vi "Blank HMI Template.vi"() -> ()   [LabVIEW 2018]
uses:
  <vilib>/NI/STM/TCP/Read Meta Data (TCP Ref).vi
  <vilib>/NI/STM/TCP/Get Connection Reference (TCP).vi
  <vilib>/NI/AMC/Read Termination Message.vi
  <vilib>/NI/AMC/Create Single Message.vi
  <vilib>/NI/AMC/Update Message Routing Info.vi
  <vilib>/NI/STM/TCP/Read Meta Data (TCP Clst).vi
  <vilib>/NI/AMC/Globals.vi
  <vilib>/NI/AMC/Send Message.vi
  <vilib>/NI/AMC/AMC.lvlib
  <vilib>/NI/STM/NI STM.lvlib
panel:
  in  "Machine":bool
  in  "Basement 4":bool
  in  "Dryer":bool
  in  "Rinse 4":bool
  in  "Rinse 3":bool
  in  "Rinse 2":bool
  in  "Basement 3":bool
  in  "Basement 2":bool
  in  "Basement 1":bool
  in  "Plater 6":bool
  in  "Plater 5":bool
  in  "Plater 4":bool
  in  "Plater 3":bool
  in  "Plater 2":bool
  in  "Plater 1":bool
  in  "Predip":bool
  in  "Rinse 1":bool
  in  "Cleaner":bool
  in  "Loader":bool
  out "status":string
  # "Module Selection"
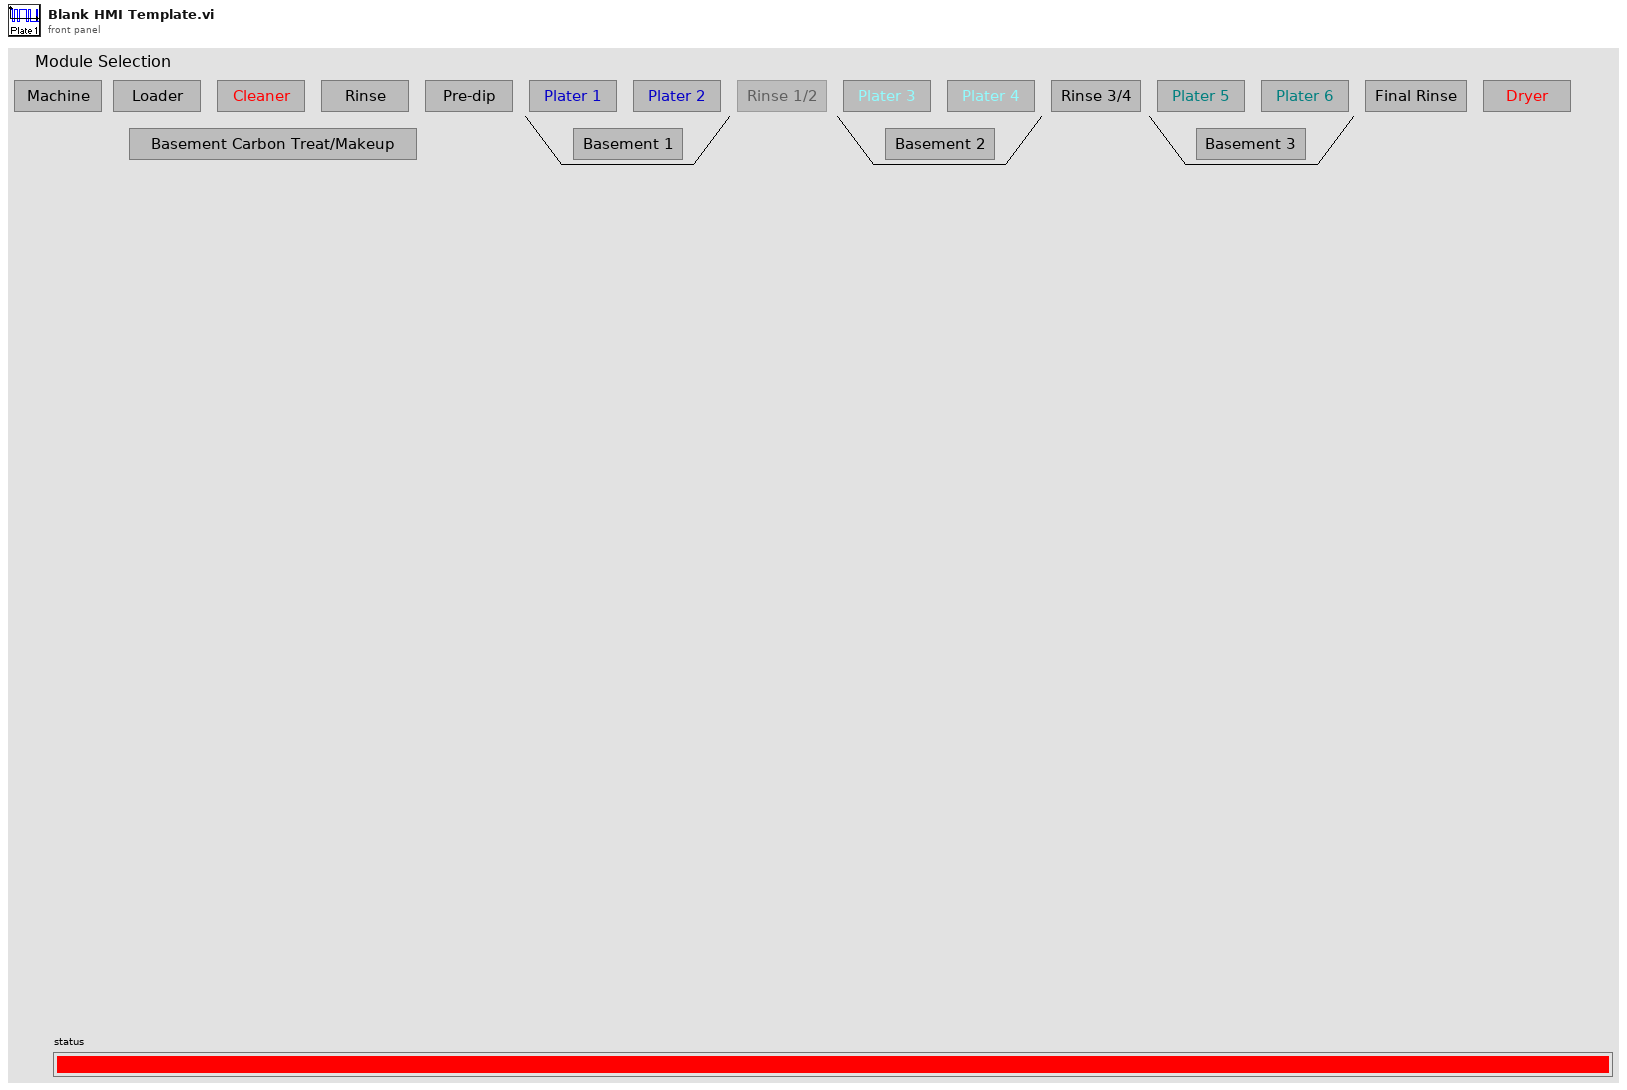
[diagram p1: front panel]
types:
  T1 = typedef "NI STM.lvlib/TCP Connection Info.ctl" = cluster{"connection ID":refnum<k5>, "meta data":T2[]}
  T2 = typedef "NI STM.lvlib/MetaDataElement.ctl" = string
  T3 = typedef "AMC.lvlib/Message Queue.ctl" = refnum<queue>
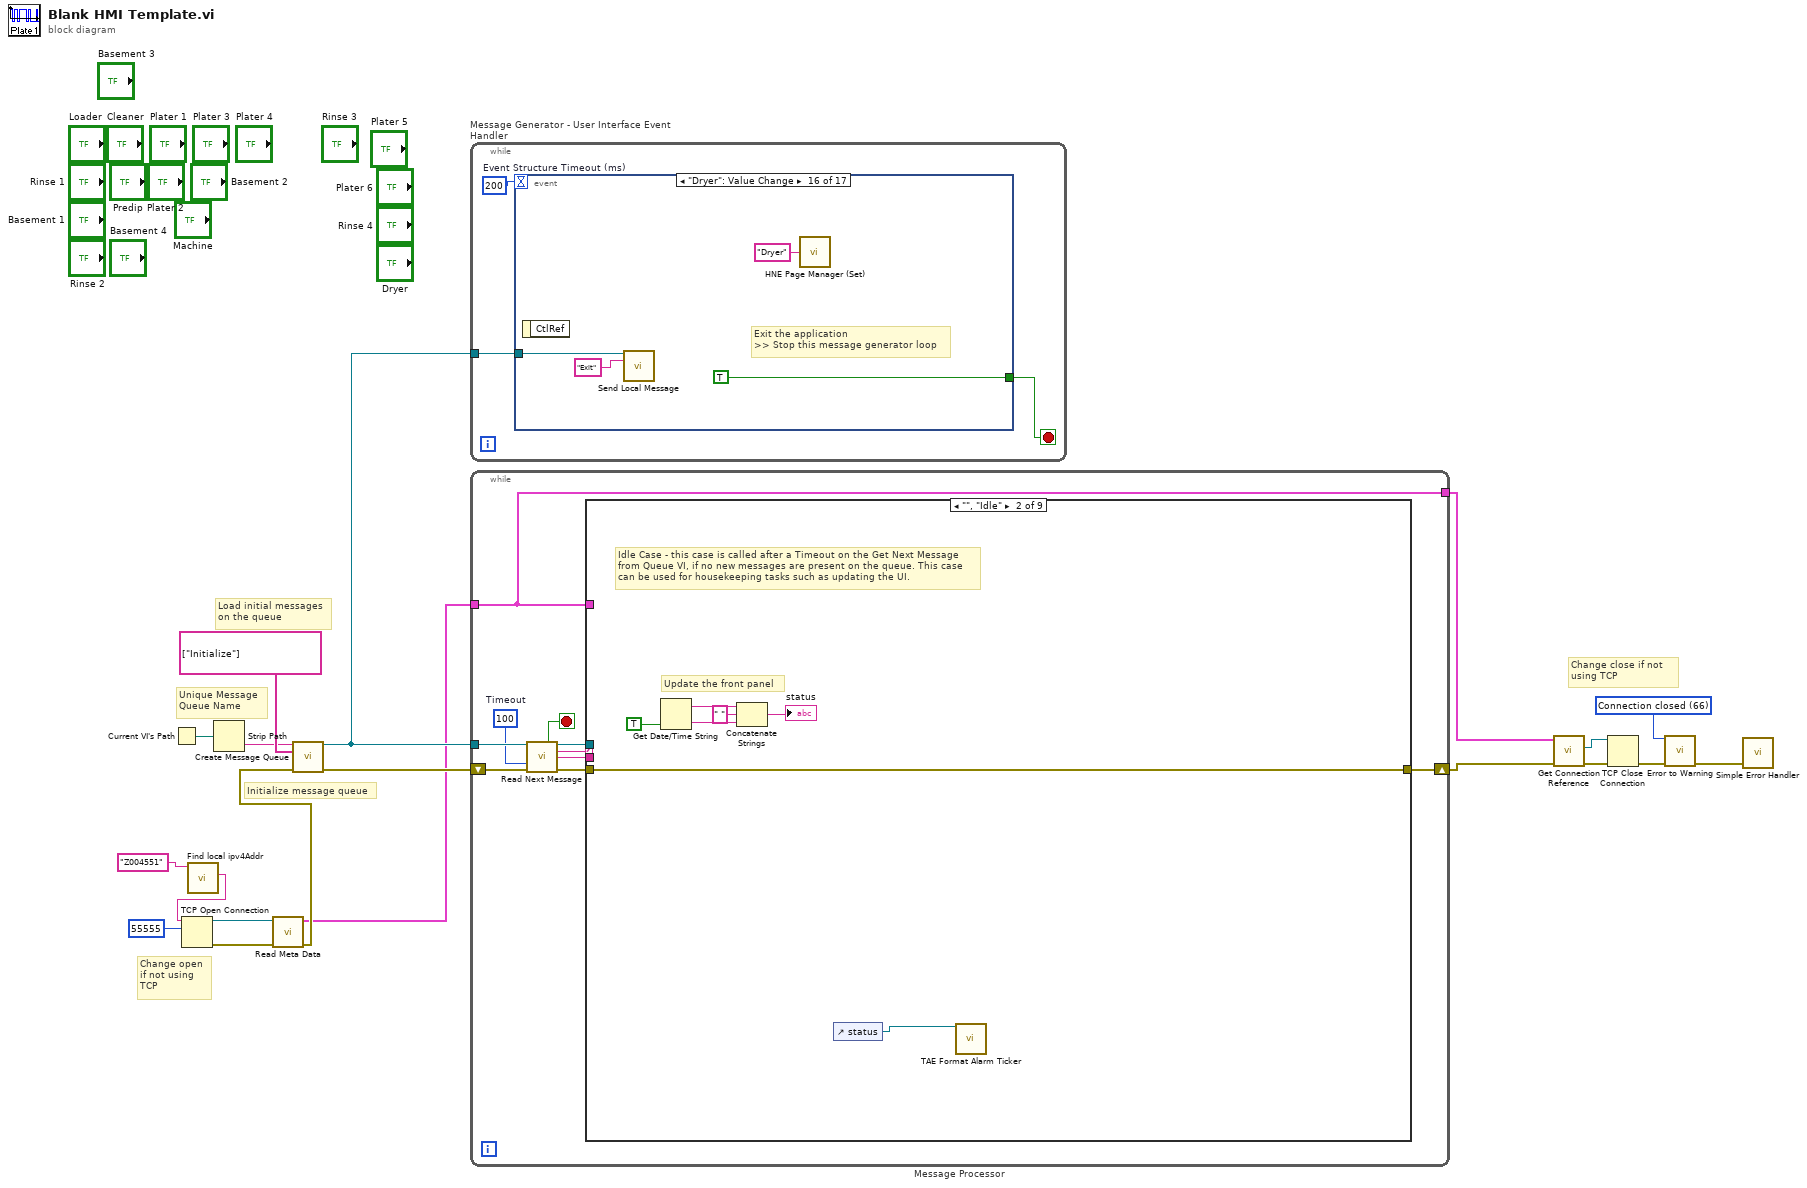
[diagram p0: block diagram]
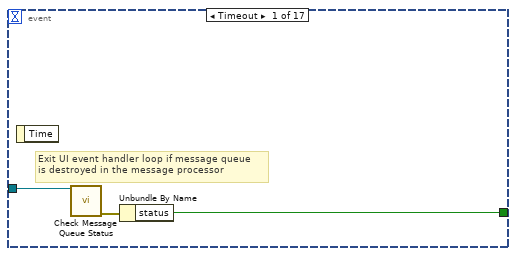
[diagram p2: hidden frame]
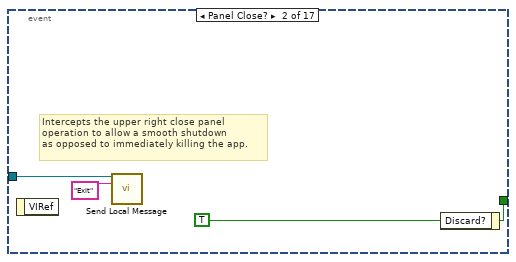
[diagram p3: hidden frame]
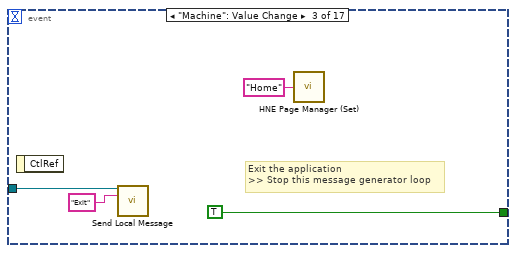
[diagram p4: hidden frame]
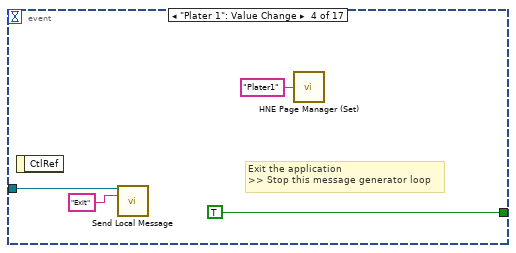
[diagram p5: hidden frame]
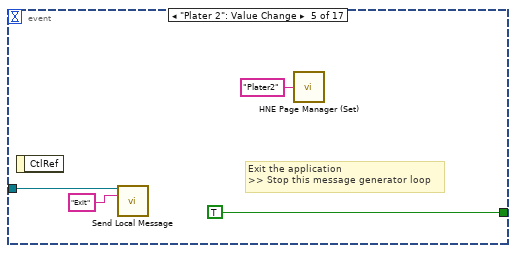
[diagram p6: hidden frame]
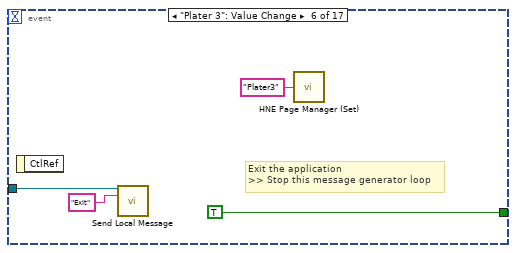
[diagram p7: hidden frame]
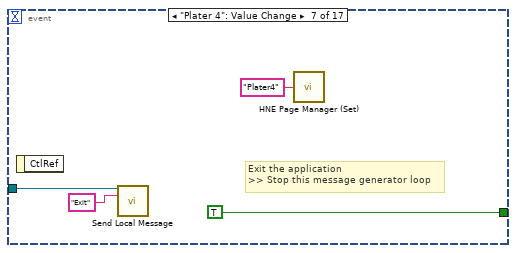
[diagram p8: hidden frame]
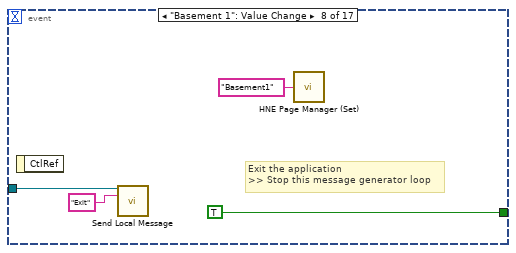
[diagram p9: hidden frame]
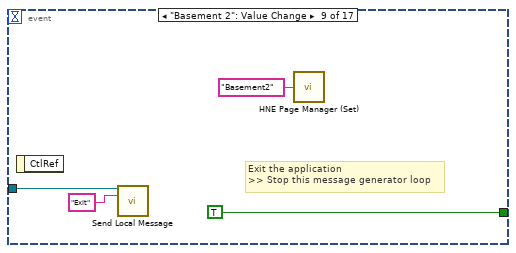
[diagram p10: hidden frame]
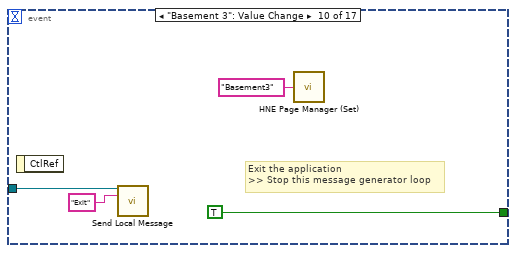
[diagram p11: hidden frame]
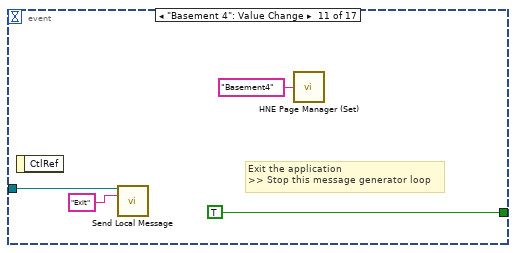
[diagram p12: hidden frame]
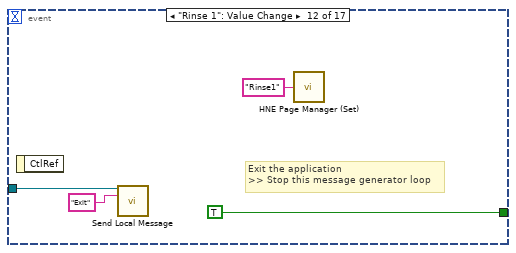
[diagram p13: hidden frame]
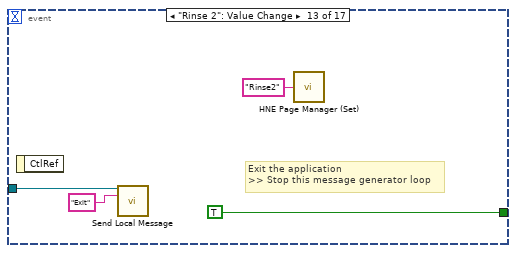
[diagram p14: hidden frame]
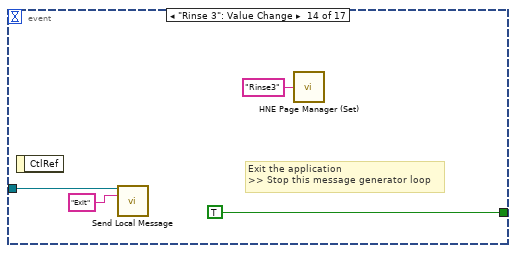
[diagram p15: hidden frame]
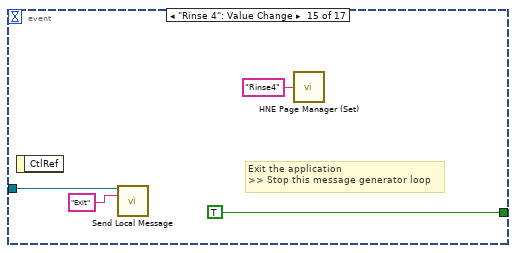
[diagram p16: hidden frame]
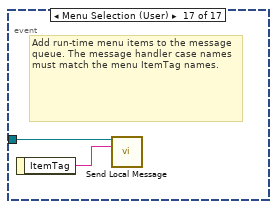
[diagram p17: hidden frame]
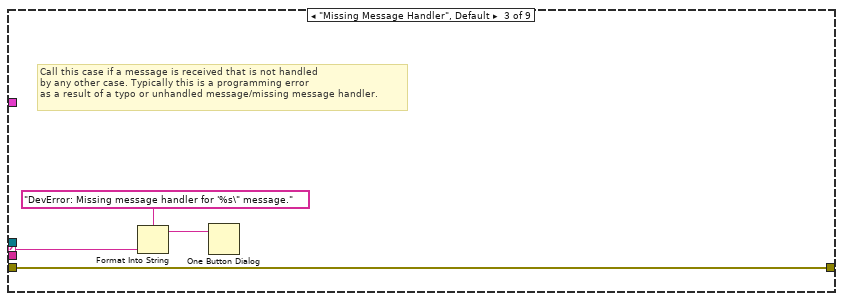
[diagram p19: hidden frame]
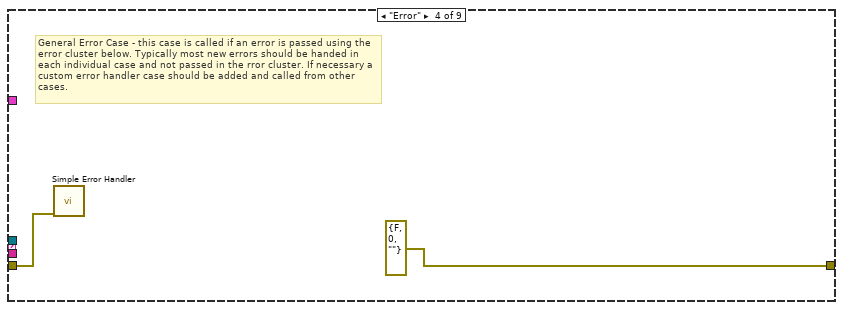
[diagram p20: hidden frame]
diagram:
  w8 = 66 items=["No Error", "Argument Error", "Memory Full", "Out of Zone", "End of File", "File Already Open", "Generic File IO Error", "File Not Found", "File Permission Error", "Disk Full", "Duplicate Path", "Too Many Files Open", "Not Enabled", "Resource File Not Found", "Cannot Add Resource", "Resource Not Found", "Image Not Found", "Image Memory Error", "Pen Does Not Exist", "Config Bad Type", "Config Token Not Found", "Config Parse Error", "Config Memory Error", "Bad External Code Format", "Bad External Code Offset", "External Code Not Present", "Null Window", "Destroy Window Mixup", "Null Menu", "Print Aborted", "Bad Print Record", "Print Driver Error", "Windows Error During Print", "Memory Error During Print", "Print Dialog Error", "Generic Print Error", "Invalid Device Refnum", "Device Not Found", "Device Parameter Error", "Device Unit Error", "Can't Open Device", "Device Call Aborted", "Generic Error", "Cancelled By User", "Object ID Too Low", "Object ID Too High", "Object Not In Heap", "Unknown Heap", "Bad DefProc ID", "DefProc Not In Table", "Message Out Of Range", "Null Method", "Unknown Message", "Manager Call Not Supported", "Bad address", "Connection In progress", "Connection timed out", "Connection is already in progress", "Network attribute not supported", "Network error", "Address in use", "System out of memory", "Connection aborted", "Connection refused", "Connection is not connected", "Connection is already connected", "Connection closed", "Initialize error (interapplication manager)", "Bad occurrence", "Wait on unbound occurrence handler", "Occurrence queue overflow", "Bad path", "Semaphore not signaled", "Unrecognized type (interapplication manager)"] ("1st Error to Convert")
  # "Change close if not using TCP"
  # "Change open if not using TCP"
  # "Initialize message queue"
  # "Unique Message\nQueue Name"
  # "Load initial messages\non the queue"
  n1 = Current VI's Path() -> (path=w15:path)
  n2 = call "Find local ipv4Addr.vi"("MachineToFind"="Z004551" ("Target IP Address")) -> ("name"=w1:string)  [unwired: 9 in, 1 out]
  n3 = TCP Open Connection(address=w1, remote port or service name=u16 55555 ("remote port")) -> (connection ID=w13:refnum<k5>, error out=w12:errorcluster)  [unwired: 1 in, 2 out]
  n4 = Strip Path(path=w15) -> (name=w18:string)  [unwired: 1 out]
  n5 = call-poly <vilib>:"Read Meta Data.vi"("error in"=w12, "connection ID"=w13) -> ("error out"=w11:errorcluster, "connection info out"=w10:T1)  [unwired: 7 in, 1 out]
  n6 = call <vilib>:"Create Message Queue.vi"("message queue name"=w18, "initial message names"=string[] ["Initialize"], "error in"=w11) -> ("message queue out"=w17:T3, "error out"=w16:errorcluster)  [unwired: 11 in]
  n7 = while "Message Generator - User Interface Event Handler" {
    tunnel: w17 -> [w20]
    stop <- w21 stop-if-true
    w22 = 200  # Event Structure Timeout (ms)
    n8 = event shown="[15] \"Dryer\": Value Change" {
      selector: _ -> [_ _ _ _ _ _ _ _ _ _ _ _ _ _ _ _ _]
      dyn-events: _ -> [_ _ _ _ _ _ _ _ _ _ _ _ _ _ _ _ _]
      timeout: w22 -> [_ _ _ _ _ _ _ _ _ _ _ _ _ _ _ _ _]
      tunnel: [w23 w28 TRUE ("Discard?") TRUE ("Discard?") TRUE ("Discard?") TRUE ("Discard?") TRUE ("Discard?") TRUE ("Discard?") TRUE ("Discard?") TRUE ("Discard?") TRUE ("Discard?") TRUE ("Discard?") TRUE ("Discard?") TRUE ("Discard?") TRUE ("Discard?") TRUE ("Discard?") _] -> w21
      tunnel: w20 -> [w24 w26 w30 w34 w38 w42 w46 w50 w54 w58 w62 w66 w70 w74 w78 w82 w85]
      event Timeout {
        # "Exit UI event handler loop if message queue\nis destroyed in the message processor"
        n9 = event-data() -> ()  [unwired: 2 out]
        n10 = call <vilib>:"Check Message Queue Status.vi"("message queue in"=w24) -> ("error out"=w25:errorcluster)  [unwired: 10 in, 4 out]
        n11 = Unbundle By Name(w25) -> ("status"=w23:bool)
      }
      event Panel Close? {
        w28 = TRUE ("Discard?")
        # "Intercepts the upper right close panel\noperation to allow a smooth shutdown\nas opposed to immediately killing the app."
        n12 = event-data() -> ()  [unwired: 2 out]
        n13 = call <vilib>:"Send Local Message.vi"("message queue in"=w26, "message name"="Exit") -> ()  [unwired: 11 in, 3 out]
        n14 = event-data("Discard?"=w28) -> ()  [unwired: 1 in, 1 out]
      }
      event "Machine": Value Change {
        # "Exit the application\n>> Stop this message generator loop"
        n15 = event-data() -> ()  [unwired: 2 out]
        n16 = call <vilib>:"Send Local Message.vi"("message queue in"=w30, "message name"="Exit") -> ()  [unwired: 11 in, 3 out]
        n17 = call <userlib>:"HNE Page Manager (Set).vi"("Next Page"="Home") -> ()  [unwired: 4 in, 1 out]
      }
      event "Plater 1": Value Change {
        # "Exit the application\n>> Stop this message generator loop"
        n18 = event-data() -> ()  [unwired: 2 out]
        n19 = call <vilib>:"Send Local Message.vi"("message queue in"=w34, "message name"="Exit") -> ()  [unwired: 11 in, 3 out]
        n20 = call <userlib>:"HNE Page Manager (Set).vi"("Next Page"="Plater1") -> ()  [unwired: 4 in, 1 out]
      }
      event "Plater 2": Value Change {
        # "Exit the application\n>> Stop this message generator loop"
        n21 = event-data() -> ()  [unwired: 2 out]
        n22 = call <vilib>:"Send Local Message.vi"("message queue in"=w38, "message name"="Exit") -> ()  [unwired: 11 in, 3 out]
        n23 = call <userlib>:"HNE Page Manager (Set).vi"("Next Page"="Plater2") -> ()  [unwired: 4 in, 1 out]
      }
      event "Plater 3": Value Change {
        # "Exit the application\n>> Stop this message generator loop"
        n24 = event-data() -> ()  [unwired: 2 out]
        n25 = call <vilib>:"Send Local Message.vi"("message queue in"=w42, "message name"="Exit") -> ()  [unwired: 11 in, 3 out]
        n26 = call <userlib>:"HNE Page Manager (Set).vi"("Next Page"="Plater3") -> ()  [unwired: 4 in, 1 out]
      }
      event "Plater 4": Value Change {
        # "Exit the application\n>> Stop this message generator loop"
        n27 = event-data() -> ()  [unwired: 2 out]
        n28 = call <vilib>:"Send Local Message.vi"("message queue in"=w46, "message name"="Exit") -> ()  [unwired: 11 in, 3 out]
        n29 = call <userlib>:"HNE Page Manager (Set).vi"("Next Page"="Plater4") -> ()  [unwired: 4 in, 1 out]
      }
      event "Basement 1": Value Change {
        # "Exit the application\n>> Stop this message generator loop"
        n30 = event-data() -> ()  [unwired: 2 out]
        n31 = call <vilib>:"Send Local Message.vi"("message queue in"=w50, "message name"="Exit") -> ()  [unwired: 11 in, 3 out]
        n32 = call <userlib>:"HNE Page Manager (Set).vi"("Next Page"="Basement1") -> ()  [unwired: 4 in, 1 out]
      }
      event "Basement 2": Value Change {
        # "Exit the application\n>> Stop this message generator loop"
        n33 = event-data() -> ()  [unwired: 2 out]
        n34 = call <vilib>:"Send Local Message.vi"("message queue in"=w54, "message name"="Exit") -> ()  [unwired: 11 in, 3 out]
        n35 = call <userlib>:"HNE Page Manager (Set).vi"("Next Page"="Basement2") -> ()  [unwired: 4 in, 1 out]
      }
      event "Basement 3": Value Change {
        # "Exit the application\n>> Stop this message generator loop"
        n36 = event-data() -> ()  [unwired: 2 out]
        n37 = call <vilib>:"Send Local Message.vi"("message queue in"=w58, "message name"="Exit") -> ()  [unwired: 11 in, 3 out]
        n38 = call <userlib>:"HNE Page Manager (Set).vi"("Next Page"="Basement3") -> ()  [unwired: 4 in, 1 out]
      }
      event "Basement 4": Value Change {
        # "Exit the application\n>> Stop this message generator loop"
        n39 = event-data() -> ()  [unwired: 2 out]
        n40 = call <vilib>:"Send Local Message.vi"("message queue in"=w62, "message name"="Exit") -> ()  [unwired: 11 in, 3 out]
        n41 = call <userlib>:"HNE Page Manager (Set).vi"("Next Page"="Basement4") -> ()  [unwired: 4 in, 1 out]
      }
      event "Rinse 1": Value Change {
        # "Exit the application\n>> Stop this message generator loop"
        n42 = event-data() -> ()  [unwired: 2 out]
        n43 = call <vilib>:"Send Local Message.vi"("message queue in"=w66, "message name"="Exit") -> ()  [unwired: 11 in, 3 out]
        n44 = call <userlib>:"HNE Page Manager (Set).vi"("Next Page"="Rinse1") -> ()  [unwired: 4 in, 1 out]
      }
      event "Rinse 2": Value Change {
        # "Exit the application\n>> Stop this message generator loop"
        n45 = event-data() -> ()  [unwired: 2 out]
        n46 = call <vilib>:"Send Local Message.vi"("message queue in"=w70, "message name"="Exit") -> ()  [unwired: 11 in, 3 out]
        n47 = call <userlib>:"HNE Page Manager (Set).vi"("Next Page"="Rinse2") -> ()  [unwired: 4 in, 1 out]
      }
      event "Rinse 3": Value Change {
        # "Exit the application\n>> Stop this message generator loop"
        n48 = event-data() -> ()  [unwired: 2 out]
        n49 = call <vilib>:"Send Local Message.vi"("message queue in"=w74, "message name"="Exit") -> ()  [unwired: 11 in, 3 out]
        n50 = call <userlib>:"HNE Page Manager (Set).vi"("Next Page"="Rinse3") -> ()  [unwired: 4 in, 1 out]
      }
      event "Rinse 4": Value Change {
        # "Exit the application\n>> Stop this message generator loop"
        n51 = event-data() -> ()  [unwired: 2 out]
        n52 = call <vilib>:"Send Local Message.vi"("message queue in"=w78, "message name"="Exit") -> ()  [unwired: 11 in, 3 out]
        n53 = call <userlib>:"HNE Page Manager (Set).vi"("Next Page"="Rinse4") -> ()  [unwired: 4 in, 1 out]
      }
      event "Dryer": Value Change {
        # "Exit the application\n>> Stop this message generator loop"
        n54 = event-data() -> ()  [unwired: 2 out]
        n55 = call <vilib>:"Send Local Message.vi"("message queue in"=w82, "message name"="Exit") -> ()  [unwired: 11 in, 3 out]
        n56 = call <userlib>:"HNE Page Manager (Set).vi"("Next Page"="Dryer") -> ()  [unwired: 4 in, 1 out]
      }
      event Menu Selection (User) {
        # "Add run-time menu items to the message\nqueue. The message handler case names must match the menu ItemTag names."
        n57 = event-data() -> ("ItemTag"=w86:string)  [unwired: 1 out]
        n58 = call <vilib>:"Send Local Message.vi"("message queue in"=w85, "message name"=w86) -> ()  [unwired: 11 in, 3 out]
      }
    }
  }
  n59 = while "Message Processor" {
    shift-left: w16 -> [w92]
    shift-right: [w96] -> w3
    tunnel: w17 -> [w93]
    tunnel: w10 -> [w87]
    tunnel: [w87] -> w4
    stop <- w95 stop-if-true
    w88 = 100  # Timeout
    n60 = call <vilib>:"Read Next Message.vi"("message queue in"=w93, "timeout (1 ms)"=w88, "error in"=w92) -> ("exit process?"=w95:bool, "message queue out"=w94:T3, "message name"=w90:string, "message value"=w89:string, "error out"=w91:errorcluster)  [unwired: 5 in, 3 out]
    n61 = case shown="\"\", \"Idle\"" w90 {
      selector: w90 -> [_ _ w107 _ _ _ _ _ _]
      tunnel: w94 -> [_ _ _ _ _ _ w114 _ _]
      tunnel: w91 -> [w97 w104 w108 w109 w111 w112 w115 w117 w122]
      tunnel: [w97 w104 w108 errorcluster {"status"=FALSE, "code"=0, "source"=""} ("error out") w111 w112 w113 w117 w122] -> w96
      tunnel: w89 -> [_ _ _ _ _ _ _ _ w121]
      tunnel: w87 -> [_ _ _ _ _ _ _ _ _]
      frame "---------- Framework Operations ----------" {
        # "Dummy case to add a seperator in the Case Structure menu"
      }
      frame "", "Idle" {
        # "Update the front panel"
        # "Idle Case - this case is called after a Timeout on the Get Next Message from Queue VI, if no new messages are present on the queue. This case can be used for housekeeping tasks such as updating the UI."
        n62 = Get Date/Time String(want seconds? (F)=TRUE) -> (date string=w103:string, time string=w102:string)  [unwired: 2 out]
        n63 = Concatenate Strings(w103, " " ("string"), w102) -> (→"status":string)
        n64 = control-ref of="status"() -> (w98:refnum<vi>)
        n65 = call <userlib>:"TAE Format Alarm Ticker.vi"("Alarm Ticker Ref"=w98) -> ()  [unwired: 15 in]
      }
      frame "Missing Message Handler", Default {
        # "Call this case if a message is received that is not handled \nby any other case. Typically this is a programming error\nas a result of a typo or unhandled message/missing message handler."
        n66 = Format Into String(format string="DevError: Missing message handler for '%s\" message." ("message"), w107) -> (resulting string=w105:string)  [unwired: 2 in, 1 out]
        n67 = One Button Dialog(message=w105) -> ()  [unwired: 2 out]
      }
      frame "Error" {
        # "General Error Case - this case is called if an error is passed using the error cluster below. Typically most new errors should be handed in each individual case and not passed in the rror cluster. If necessary a custom error handler case should be added and called from other cases."
        n68 = call <vilib>:"Simple Error Handler.vi"("error in (no error)"=w109) -> ()  [unwired: 1 in, 8 out]
      }
      frame "---------- Generic Operations ----------" {
        # "Dummy case to add a seperator in the Case Structure menu"
      }
      frame "Initialize" {
        # "Initialize the state variables and user interface"
      }
      frame "Exit" {
        # "Destroy message queue >> this will halt the UI event handler loop"
        # "Stop the VI\n>> Perform any cleanup tasks in this message case.\n>> Clear display before closing."
        n69 = call <vilib>:"Destroy Message Queue.vi"("message queue in"=w114, "error in"=w115) -> ("error out"=w113:errorcluster)  [unwired: 11 in, 2 out]
        n70 = local write "status"("" ("Status")) -> ()
      }
      frame "---------- Application Operations ----------" {
        # "Dummy case to add a seperator in the Case Structure menu"
      }
      frame "Process Data" {
        # "Add actions to perform in response to Process button being pressed"
        n71 = Fract/Exp String To Number(string=w121) -> (number=w120:dbl)  [unwired: 4 out]
        n72 = Format Into String(format string="Process Data: %f" ("message"), w120) -> (resulting string=w118:string)  [unwired: 2 in, 1 out]
        n73 = One Button Dialog(message=w118) -> ()  [unwired: 2 out]
      }
    }
  }
  n74 = call-poly <vilib>:"Get Connection Reference.vi"("error in"=w3, "connection info in"=w4) -> ("error out"=w7:errorcluster, "connection ID out"=w6:refnum<k5>)  [unwired: 8 out]
  n75 = TCP Close Connection(connection ID=w6, error in (no error)=w7) -> (error out=w9:errorcluster)  [unwired: 2 out]
  n76 = call <vilib>:"Error to Warning.vi"("1st Error to Convert"=w8, "error in"=w9) -> ("warning out"=w5:errorcluster)  [unwired: 3 in, 10 out]
  n77 = call <vilib>:"Simple Error Handler.vi"("error in (no error)"=w5) -> ()  [unwired: 4 in, 5 out]
